vi "Set Amplitude.vi"(8 "error in (no error)":errorcluster, 10 "Output amplitude":dbl=1.0 min=-1.0 max=1.0 format="%#_8pV", 11 "Lock-in Driver in":refnum<class "Lock-in Driver.lvclass">) -> (0 "error out":errorcluster, 3 "Lock-in Driver out":refnum<class "Lock-in Driver.lvclass">)   [LabVIEW 2021, in "Lock-in Driver.lvclass"]
uses:
  Lock-in Driver.lvclass
  Lock-in Driver.lvclass/Lock-in Driver.ctl
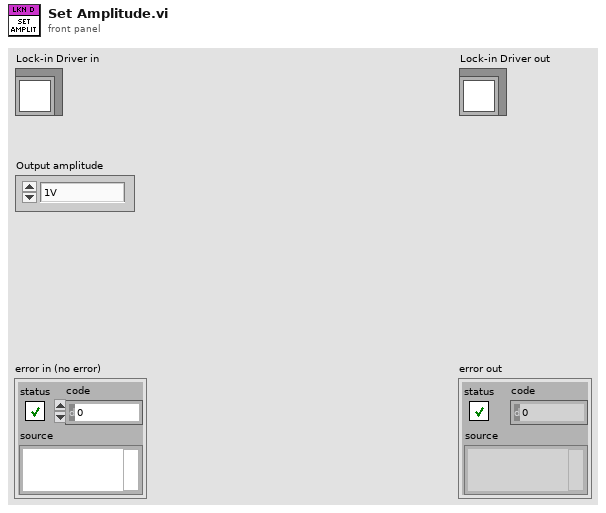
[diagram p1: front panel]
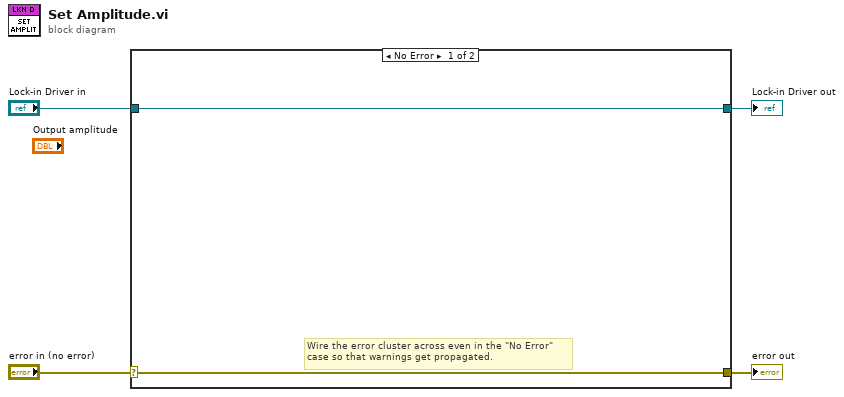
[diagram p0: block diagram]
diagram:
  n1 = case shown="No Error" "error in (no error)" {
    selector: "error in (no error)" -> [w5 w8]
    tunnel: [w5 w8] -> w3
    tunnel: [w6 w7] -> w1
    tunnel: "Lock-in Driver in" -> [w6 w7]
    frame No Error {
      # "Wire the error cluster across even in the \"No Error\"\ncase so that warnings get propagated."
    }
    frame Error {
    }
  }
  "error out" <- w3
  "Lock-in Driver out" <- w1
